vi "OSP.vi"() -> ()   [LabVIEW 2019]
uses:
  <vilib>/vision/NI_Vision_Development_Module.lvlib
panel:
  out "String (OCR/OCV 2)":string
  out "Image":T1(plugin-control)
  out "return value 3":i32[](array[numeric])
  in  "Path Control":path
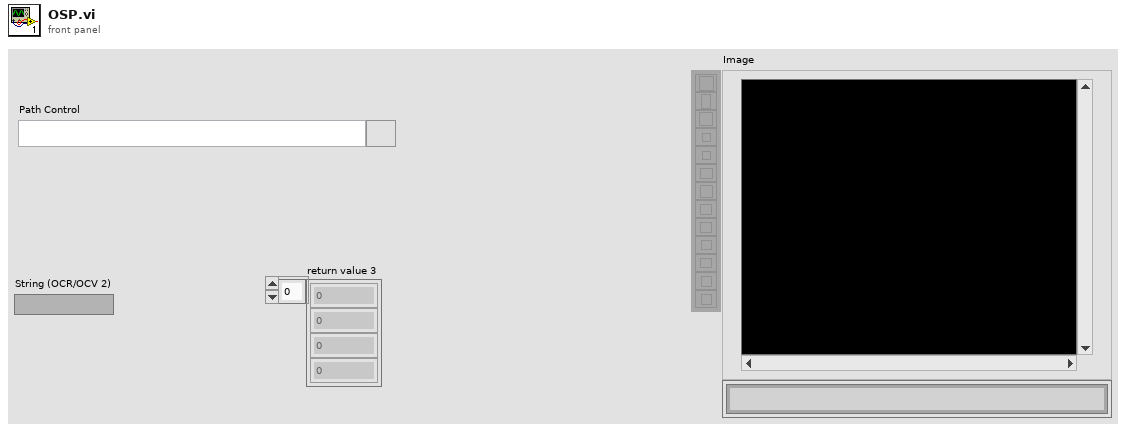
[diagram p1: front panel]
types:
  T1 = typedef "IMAQ Image.ctl" = refnum<image>
  T2 = typedef "Image Type" = u32
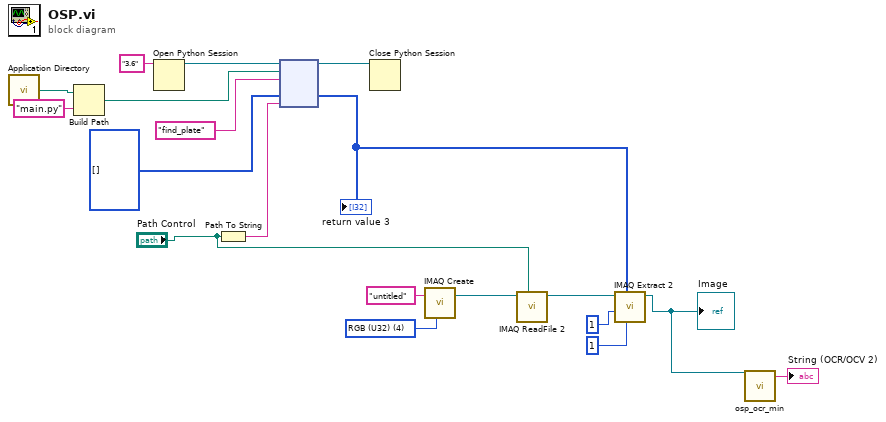
[diagram p0: block diagram]
diagram:
  w9 = T2 4 items=["Grayscale (U8)", "Grayscale (I16)", "Grayscale (SGL)", "Complex (CSG)", "RGB (U32)", "HSL (U32)", "RGB (U64)", "Grayscale (U16)"] ("Image Type")
  n1 = call <vilib>:"Application Directory.vi"() -> ("Application Directory"=w13:path)
  n2 = Build Path(base path=w13, name or relative path="main.py") -> (appended path=w11:path)
  n3 = Open Python Session(python version="3.6" ("Python version")) -> (session out=w18:refnum<k35>)  [unwired: 2 in, 1 out]
  n4 = Path To String(path="Path Control") -> (string=w15:string)
  n5 = node(w18, w11, "find_plate" ("function name"), i32[] [], w15) -> (w17:refnum<k35>, w3:i32[])  [unwired: 2 in, 3 out]
  "return value 3" <- w3
  n6 = Close Python Session(session in=w17) -> ()  [unwired: 1 in, 1 out]
  n7 = call "IMAQ Create"("Image Name"="untitled", "Image Type"=w9) -> ("New Image"=w8:T1)  [unwired: 3 in, 1 out]
  n8 = call "IMAQ ReadFile 2"("File Path"="Path Control", "Image"=w8) -> ("Image Out"=w6:T1)  [unwired: 5 in, 4 out]
  n9 = call "IMAQ Extract 2"("Y Step Size"=1, "Optional Rectangle"=w3, "X Step Size"=1, "Image Src"=w6) -> ("Image Dst Out"=w2:T1)  [unwired: 6 in, 1 out]
  "Image" <- w2
  n10 = call "osp_ocr_min.vi"("Image In"=w2) -> ("String (OCR/OCV 2)"=→"String (OCR/OCV 2)":string)  [unwired: 24 in, 2 out]
